vi "GetIdentityAttr.vi"(8 "error in (no error)":errorcluster, 11 "SMO in":refnum<class "SMO.lvclass">) -> (0 "error out":errorcluster, 2 "Attribute.Identity":refnum<class "Attribute.Identity.lvclass">, 3 "SMO out":refnum<class "SMO.lvclass">)   [LabVIEW 2013, in "SMO.lvclass"]
uses:
  SMO.lvclass
  Support/Attribute.Identity/Attribute.Identity.lvclass
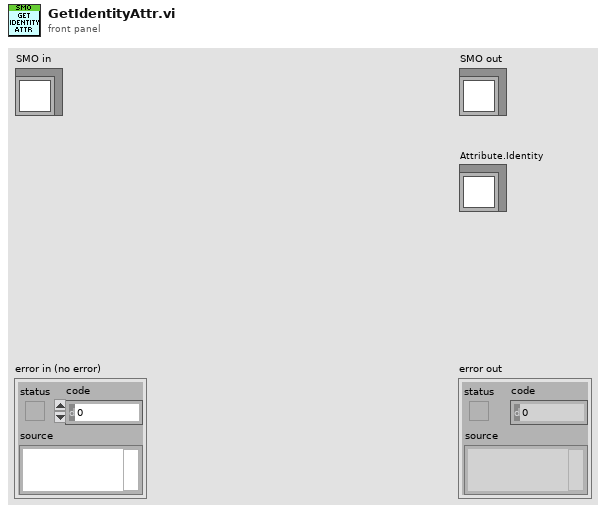
[diagram p1: front panel]
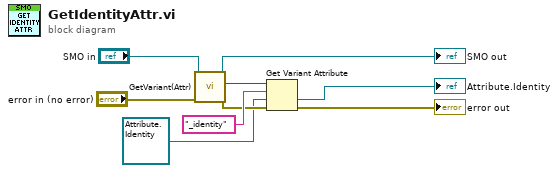
[diagram p0: block diagram]
diagram:
  n1 = call "GetVariant(Attr).vi"("error in (no error)"="error in (no error)", "SMO in"="SMO in") -> ("error out"=w7:errorcluster, "[Attributes]"=w9:variant, "SMO out"=→"SMO out":refnum<class "SMO.lvclass">)  [unwired: 7 in]
  n2 = Get Variant Attribute(Variant=w9, name="_identity", default value (empty Variant)=refnum<class "Attribute.Identity.lvclass"> refnum, error in=w7) -> (value=→"Attribute.Identity":refnum<class "Attribute.Identity.lvclass">, error out=→"error out":errorcluster)  [unwired: 2 out]
